vi "battery_logger.vi"() -> ()   [LabVIEW 2017]
uses:
  <vilib>/Utility/error.llb/whitespace.ctl
  <vilib>/Analysis/baseanly.llb/Mean (DBL).vi
  <vilib>/Analysis/NI_AALBase.lvlib
panel:
  out "Array":dbl[](array[numeric])
  out "Corriente":dbl
  out "Corriente":dbl(graph) caption="Waveform Chart"
  out "Tensión (V)":dbl
  out "S1":dbl(graph) caption="Waveform Chart"
  in  "stop (F)":bool
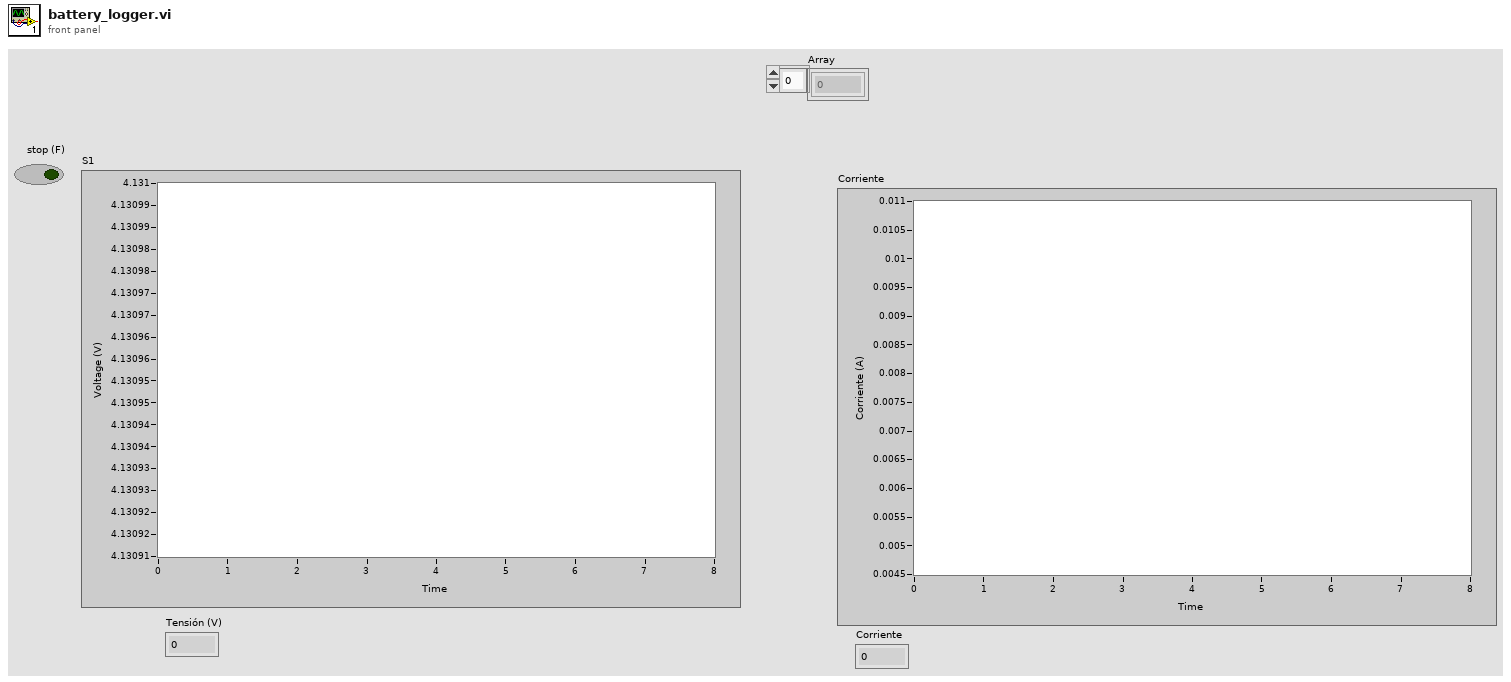
[diagram p1: front panel]
types:
  T1 = enum16{"open", "open or create", "create or replace", "create", "open (read only)"}
  T2 = typedef "whitespace.ctl" = u16
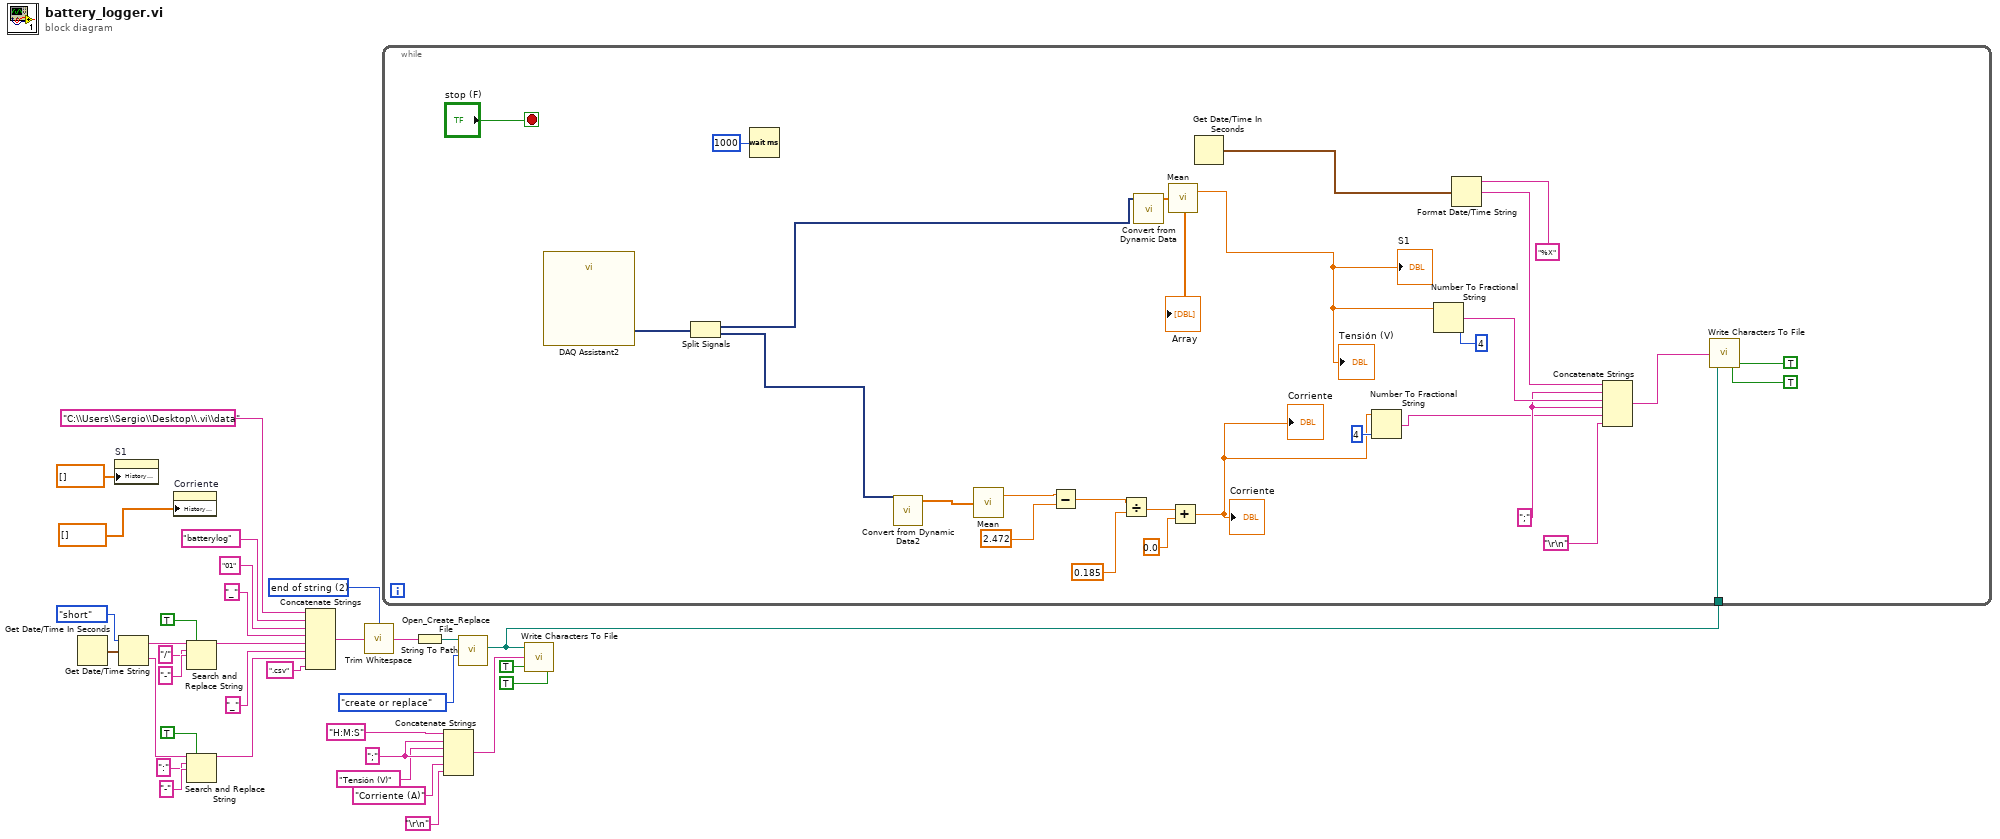
[diagram p0: block diagram]
diagram:
  w8 = ";"
  w18 = T2 2 items=["both", "start of string", "end of string"] ("location (both)")
  n1 = Get Date/Time In Seconds() -> (seconds since 1Jan1904=w20:timestamp)
  n2 = property on="S1" class="WFChart (strict)"("History Data"=dbl[] []) -> ()  [unwired: 2 in, 2 out]
  n3 = Get Date/Time String(date format (0)=enum16{"short", "long", "abbreviated"}."short", seconds (now)=w20) -> (date string=w22:string, time string=w29:string)  [unwired: 1 in]
  n4 = property on="Corriente" class="WFChart (strict)"("History Data"=dbl[] []) -> ()  [unwired: 2 in, 2 out]
  n5 = Search and Replace String(replace all?=TRUE ("replace all? (F)"), input string=w22, search string="/", replace string="-" ("replace string (\"\")")) -> (result string=w26:string)  [unwired: 4 in, 3 out]
  n6 = Search and Replace String(replace all?=TRUE ("replace all? (F)"), input string=w29, search string=":", replace string="-" ("replace string (\"\")")) -> (result string=w32:string)  [unwired: 4 in, 3 out]
  n7 = Concatenate Strings("C:\\Users\\Sergio\\Desktop\\.vi\\data" ("string"), "batterylog" ("string"), "01" ("string"), "_" ("string"), w26, "_" ("string"), w32, ".csv" ("string")) -> (w19:string)
  n8 = call <vilib>:"Trim Whitespace.vi"("string"=w19, "location (both)"=w18) -> ("trimmed string"=w11:string)
  n9 = String To Path(string=w11) -> (path=w14:path)
  n10 = Concatenate Strings("H:M:S" ("文字列"), w8, "Tensión (V)" ("文字列"), w8, "Corriente (A)" ("string"), "\r\n") -> (w5:string)
  n11 = call <vilib>:"Open_Create_Replace File.vi"("function (open:0)"=T1."create or replace", "file path"=w14) -> ("new file path"=w2:path)  [unwired: 6 in, 3 out]
  n12 = while {
    tunnel: w2 -> [w54]
    stop <- "stop (F)" stop-if-true
    w51 = ";"
    n13 = call "DAQ Assistant2"() -> ("data"=w46:dynamicdata)  [unwired: 16 in, 3 out]
    n14 = Split Signals(w46) -> (w45:dynamicdata, w38:dynamicdata)  [unwired: 2 in]
    n15 = Wait (ms)(milliseconds to wait=u32 1000) -> ()  [unwired: 1 out]
    n16 = call "Convert from Dynamic Data2"("Dynamic Data Type"=w38) -> ("Array"=w42:dbl[])  [unwired: 3 in]
    n17 = call-poly <vilib>:"Mean.vi"("X"=w42) -> ("mean"=w41:dbl)  [unwired: 1 out]
    n18 = Subtract(x=w41, y=2.472) -> (x-y=w39:dbl)
    n19 = Divide(x=w39, y=0.185) -> (x/y=w37:dbl)
    n20 = call "Convert from Dynamic Data"("Dynamic Data Type"=w45) -> ("Array"=w44:dbl[])  [unwired: 3 in]
    "Array" <- w44
    n21 = call-poly <vilib>:"Mean.vi"("X"=w44) -> ("mean"=w52:dbl)  [unwired: 1 out]
    "S1" <- w52
    "Tensión (V)" <- w52
    n22 = Add(x=w37, y=0.0) -> (x+y=w36:dbl)
    "Corriente" <- w36
    "Corriente" <- w36
    n23 = Get Date/Time In Seconds() -> (seconds since 1Jan1904=w55:timestamp)
    n24 = Number To Fractional String(number=w36, precision (6)=i16 4) -> (F-format string=w49:string)  [unwired: 2 in]
    n25 = Number To Fractional String(number=w52, precision (6)=i16 4) -> (F-format string=w62:string)  [unwired: 2 in]
    n26 = Format Date/Time String(time format string (%c)="%X", seconds (now)=w55) -> (date/time string=w60:string)  [unwired: 1 in]
    n27 = Concatenate Strings(w60, w51, w62, w51, w49, "\r\n") -> (w58:string)
    n28 = call <vilib>:"Write Characters To File.vi"("convert eol? (no:F)"=TRUE, "append to file? (new file:F)"=TRUE, "character string"=w58, "file path (dialog if empty)"=w54) -> ()  [unwired: 1 in, 1 out]
  }
  n29 = call <vilib>:"Write Characters To File.vi"("convert eol? (no:F)"=TRUE, "append to file? (new file:F)"=TRUE, "character string"=w5, "file path (dialog if empty)"=w2) -> ()  [unwired: 1 in, 1 out]
